vi "UTIL_OpenVectorFile_Debug.vi"() -> (0 "error out":errorcluster, 1 "Numeric":i32, 2 "path":path, 3 "before match":string, 4 "data 2":dbl[][](array[numeric]), 5 "data":dbl[](array[numeric]))   [LabVIEW 2024]
uses:
  <vilib>/Utility/NIReport.llb/Report Type.ctl
  <vilib>/addons/_office/excel.llb/Excel Get Data ([dbl]).vi
  <vilib>/regexp/Match Regular Expression.xnode
  <vilib>/Utility/NIReport.llb/NI_report.lvclass
  <vilib>/Utility/NIReport.llb/Excel/NI_Excel.lvclass
  <vilib>/addons/_office/NI_ReportGenerationToolkit.lvlib
  <vilib>/Utility/NIReport.llb/NI_ReportGenerationCore.lvlib
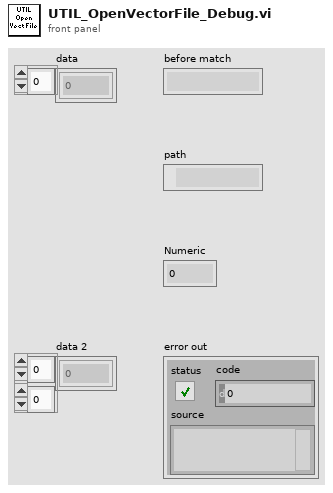
[diagram p1: front panel]
types:
  T1 = typedef "NI_ReportGenerationCore.lvlib/Report Type.ctl" = enum16{"HTML", "Word", "Excel"}
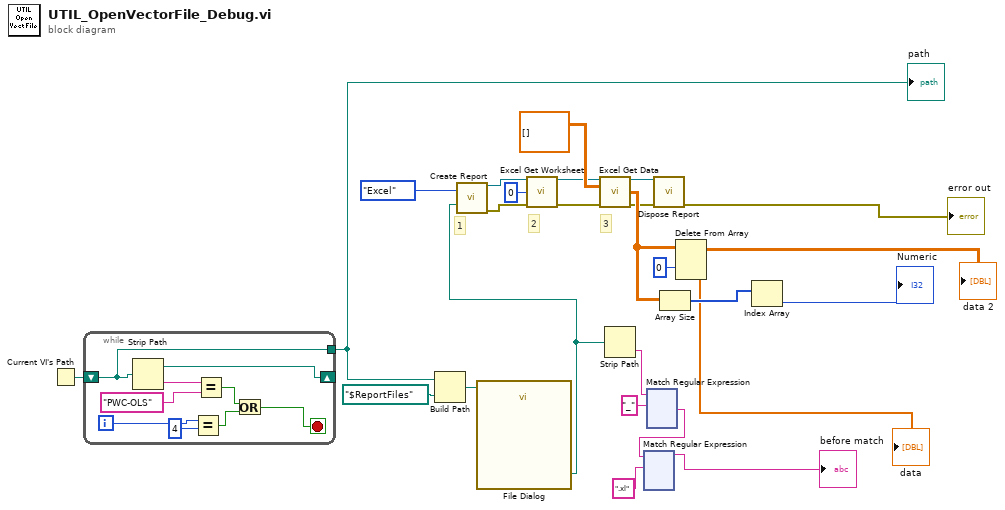
[diagram p0: block diagram]
diagram:
  # "3"
  # "2"
  # "1"
  n1 = Current VI's Path() -> (path=w11:path)
  n2 = while {
    shift-right: [w28] -> _
    shift-left: w11 -> [w27]
    tunnel: [w27] -> w17
    i -> [w33]
    stop <- w29 stop-if-true
    n3 = Strip Path(path=w27) -> (stripped path=w28:path, name=w34:string)
    n4 = Equal?(x=w33, y=4) -> (x = y?=w30:bool)
    n5 = Equal?(x=w34, y="PWC-OLS") -> (x = y?=w31:bool)
    n6 = Or(x=w31, y=w30) -> (x .or. y?=w29:bool)
  }
  "path" <- w17
  n7 = Build Path(base path=w17, name or relative path=path "$ReportFiles" ("name or relative path 2")) -> (appended path=w13:path)
  n8 = call "File Dialog"("start path"=w13) -> ("selected path"=w20:path)  [unwired: 11 in, 3 out]
  n9 = call <vilib>:"Create Report.vi"("report type"=Report_Type."Excel", "template (empty)"=w20) -> ("report out"=w5:refnum<class "NI_report.lvclass">, "error out"=w6:errorcluster)  [unwired: 12 in]
  n10 = call <vilib>:"Excel Get Worksheet.vi"("report in"=w5, "worksheet index (0)"=0, "error in (no error)"=w6) -> ("report out"=w3:refnum<class "NI_report.lvclass">, "error out"=w2:errorcluster)  [unwired: 11 in]
  n11 = call-poly <vilib>:"Excel Get Data.vi"("report in"=w3, "data type"=dbl[][] [], "error in (no error)"=w2) -> ("report out"=w19:refnum<class "NI_report.lvclass">, "data"=w14:dbl[][], "error out"=w9:errorcluster)  [unwired: 10 in]
  n12 = Strip Path(path=w20) -> (name=w24:string)  [unwired: 1 out]
  n13 = xnode "Match Regular Expression"("input string"=w24, "regular expression"="_") -> ("after match"=w25:string)  [unwired: 4 in, 4 out]
  n14 = xnode "Match Regular Expression"("input string"=w25, "regular expression"=".xl") -> ("before match"=→"before match":string)  [unwired: 4 in, 4 out]
  n15 = call-dynamic "Dispose Report.vi"("report in"=w19, "error in (no error)"=w9) -> ("error out"=→"error out":errorcluster)  [unwired: 13 in]
  n16 = Array Size(array=w14) -> (size(s)=w26:i32[])
  n17 = Delete From Array(array=w14, index (row)=0) -> (deleted portion=→"data":dbl[], array with subset deleted=→"data 2":dbl[][])  [unwired: 2 in]
  n18 = Index Array(array=w26) -> (element=→"Numeric":i32)  [unwired: 1 in]
